vi "SGUI Global Var.vi"() -> ()   [LabVIEW 2020, in "varilib.lvlib"]
uses:
  varilib.lvlib
panel:
  in  "ctrl groups stack":T1(array[cluster])
  in  "labels":string[](array[string])
  in  "ctrl refs":refnum<vi>[](array[refnum])
  in  "ctrl list":T2(array[cluster])
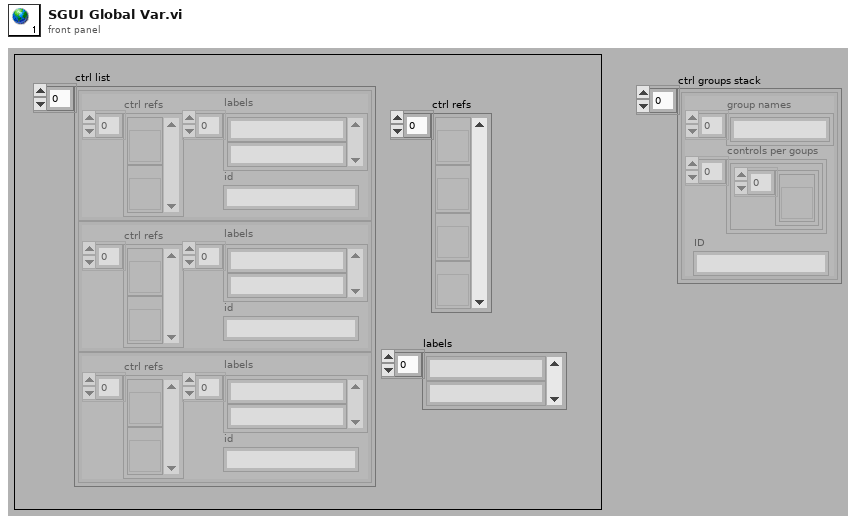
[diagram p1: front panel]
types:
  T1 = cluster{"group names":string[], "controls per goups":cluster{"control references (empty)":refnum<vi>[]}[], "ID":string}[]
  T2 = cluster{"ctrl refs":refnum<vi>[], "labels":string[], "id":string}[]
diagram:
